vi "Clock Check.vi"() -> ()   [LabVIEW 2019]
uses:
  <vilib>/Platform/TimedLoop/XDataNode/timing_clust.ctl
  <vilib>/Platform/TimedLoop/XDataNode/nitl_modes.ctl
  <vilib>/Platform/TimedLoop/XDataNode/wakeup.ctl
  <vilib>/rvi/Emulation/niFpgaSctlEmulationGetInTimedLoop.vi
  <vilib>/rvi/Emulation/niFpgaEmulationReportErrorSimple.vi
  <vilib>/rvi/Emulation/niFpgaGetClockAttributes.vi
  <vilib>/rvi/Emulation/niFpgaCriticalErrorInLSC.vi
  P:/Jeff R/FPGA Global.vi
  <vilib>/rvi/eio/common/nirviEmuTemplateMethod_errors.vi
  <vilib>/platform/TimedLoop/XDataNode/XDataNode.xnode
  <vilib>/eio/EIONode/EIONode.xnode
  <vilib>/eio/EIOMethodNode/EIOMethodNode.xnode
  <vilib>/Platform/TimedLoop/XDataNode/XDNodeRunTimeDep.lvlib
panel:
  in  "Frequency":T1(ring)
  in  "Square Wave":bool caption="Output on\nConn 2/ DIO0"
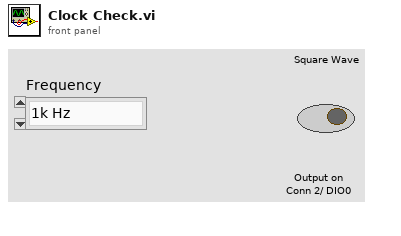
[diagram p1: front panel]
types:
  T1 = enum16{"1k Hz", "10k Hz", "100k Hz", "1M Hz", "10M Hz"}
  T2 = typedef "XDNodeRunTimeDep.lvlib/timing_clust.ctl" = cluster{"Expected End [f-1]":u64, "Actual End [f-1]":u64, "Finished Late? [f-1]":bool, "Expected End [i-1]":u64, "Actual End [i-1]":u64, "Finished Late? [i-1]":bool, "Expected Start [i]":u64, "Actual Start [i]":u64, "Expected Start [f]":u64, "Actual Start [f]":u64, "Source Name":string, "Structure Name":string, "Period":i64, "Deadline":i64, "Offset":i64, "Start":i64, "Priority":i32, "Timeout":i32, "Mode":T3, "Wakeup Reason":T4, "Error":errorcluster, "Source Type":string, "Secondary Source Type":string, "Global End Time":u64, "Global Start Time":u64, "Frame Duration":u64, "Iteration Duration":u64, "Assigned CPU":i32, "I/O Scan Engine Mode":u32}
  T3 = typedef "XDNodeRunTimeDep.lvlib/nitl_modes.ctl" = enum32{"No Change", "Process missed periods, maintain original phase", "Discard missed periods, maintain original phase", "Process missed periods, ignore original phase", "Discard missed periods, ignore original phase"}
  T4 = typedef "XDNodeRunTimeDep.lvlib/wakeup.ctl" = enum32{"Normal", "Aborted", "Asynchronous wakeup", "Timing source error", "Timed loop error", "Timeout"}
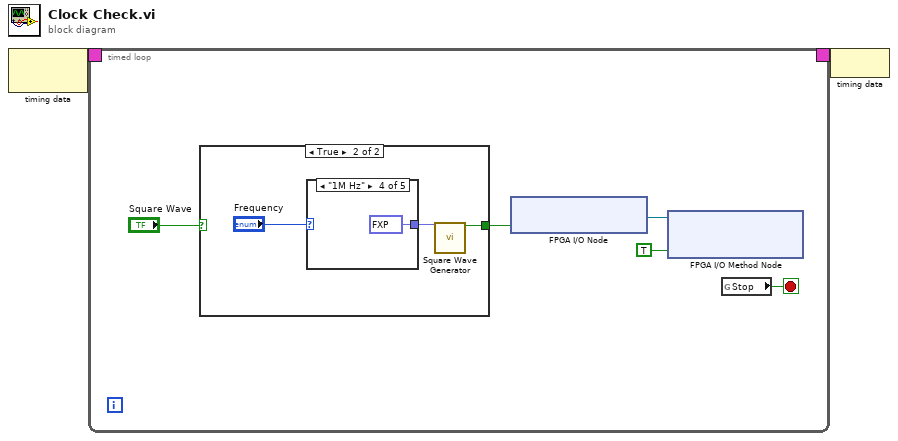
[diagram p0: block diagram]
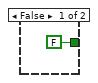
[diagram p2: hidden frame]
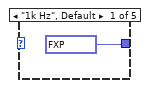
[diagram p3: hidden frame]
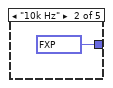
[diagram p4: hidden frame]
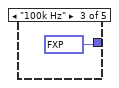
[diagram p5: hidden frame]
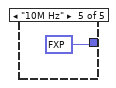
[diagram p6: hidden frame]
diagram:
  n1 = node-c288() -> (w2:T2)  [unwired: 1 in]
  n2 = timed-loop "Timed Loop" {
    timing: w2 -> [_]
    timing-out: [_] -> w1
    stop <- w7 stop-if-true
    n3 = case shown="True" "Square Wave" {
      tunnel: [FALSE ("square wave out") w9] -> w4
      frame False {
      }
      frame True {
        n4 = case shown="\"1M Hz\"" "Frequency" {
          tunnel: [fxp<+,32,0> 2.4999957531690598e-05 ("frequency (periods/tick)") fxp<+,32,0> 0.0002500000409781933 ("frequency (periods/tick)") fxp<+,32,0> 0.0024999999441206455 ("frequency (periods/tick)") fxp<+,32,0> 0.024999999906867743 ("frequency (periods/tick)") fxp<+,32,0> 0.25 ("frequency (periods/tick)")] -> w10
          frame "1k Hz", Default {
          }
          frame "10k Hz" {
          }
          frame "100k Hz" {
          }
          frame "1M Hz" {
          }
          frame "10M Hz" {
          }
        }
        n5 = call "Square Wave Generator"("frequency (periods/tick)"=w10) -> ("square wave out"=w9:bool)  [unwired: 14 in]
      }
    }
    n6 = xnode "FPGA I/O Node"("Connector2/DIO0"=w4) -> ("FPGA I/O Out"=w5:refnum<k21>)  [unwired: 1 in]
    n7 = xnode "FPGA I/O Method Node"("FPGA I/O In"=w5, "Enable"=TRUE) -> ()  [unwired: 1 out]
    n8 = global read "FPGA Global.vi" "Stop"() -> (w7:bool)
  }
  n9 = node-c288(w1) -> ()
